vi "PID Control.vi"(0 "Set Point":cluster{"SetPoint X":dbl, "SetPoint Y":dbl}, 3 "Actual Value":cluster{"Actual X":dbl, "Actual Y":dbl}, 4 "PID Gain X":T1={"proportional gain (Kc)"=1.0, "integral time (Ti, min)"=0.01, "derivative time (Td, min)"=0.0} {"derivative time (Td, min)" format="%.3f"; "integral time (Ti, min)" format="%.3f"; "proportional gain (Kc)" format="%.3f"}, 5 "PID Gain Y":T1={"proportional gain (Kc)"=1.0, "integral time (Ti, min)"=0.01, "derivative time (Td, min)"=0.0} {"derivative time (Td, min)" format="%.3f"; "integral time (Ti, min)" format="%.3f"; "proportional gain (Kc)" format="%.3f"}) -> (7 "Output PID X":dbl format="%.2f", 10 "Output PID Y":dbl format="%.2f")   [LabVIEW 2015]
uses:
  <vilib>/addons/control/pid/pid.llb/PID (DBL).vi
  <vilib>/addons/control/pid/NI_PID_pid.lvlib
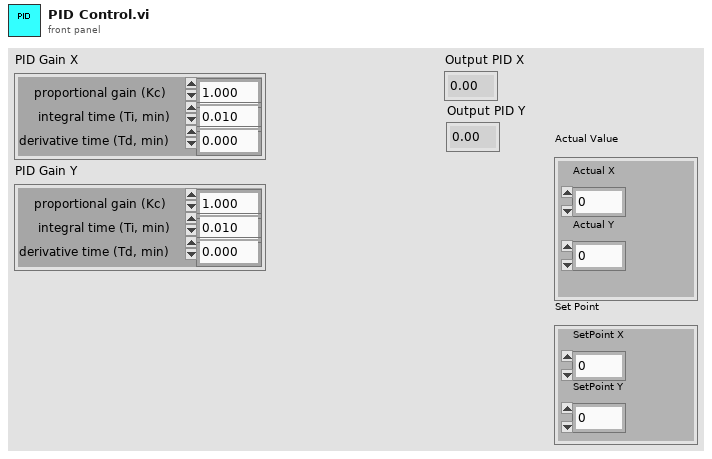
[diagram p1: front panel]
types:
  T1 = cluster{"proportional gain (Kc)":dbl, "integral time (Ti, min)":dbl, "derivative time (Td, min)":dbl}
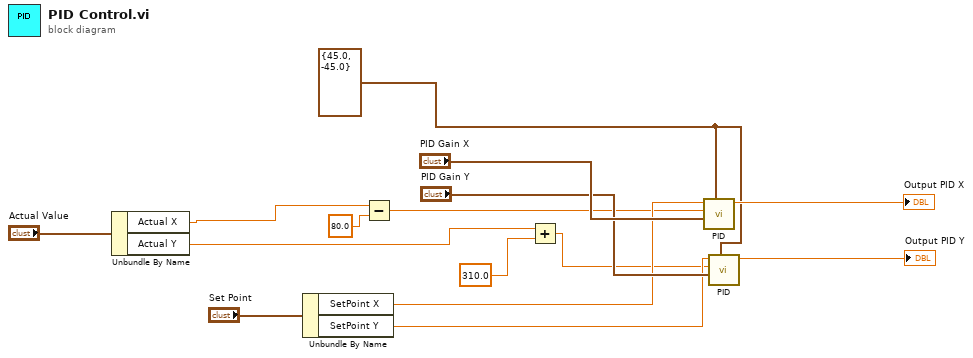
[diagram p0: block diagram]
diagram:
  w1 = cluster{dbl, dbl} {45.0, -45.0}
  n1 = Unbundle By Name("Actual Value") -> ("Actual X"=w7:dbl, "Actual Y"=w5:dbl)
  n2 = Unbundle By Name("Set Point") -> ("SetPoint X"=w11:dbl, "SetPoint Y"=w10:dbl)
  n3 = Subtract(x=w7, y=80.0) -> (x-y=w6:dbl)
  n4 = Add(x=w5, y=310.0) -> (x+y=w4:dbl)
  n5 = call-poly <vilib>:"PID.vi"("output range"=w1, "PID gains"="PID Gain X", "process variable"=w6, "setpoint"=w11) -> ("output"=→"Output PID X":dbl)  [unwired: 6 in, 1 out]
  n6 = call-poly <vilib>:"PID.vi"("output range"=w1, "PID gains"="PID Gain Y", "process variable"=w4, "setpoint"=w10) -> ("output"=→"Output PID Y":dbl)  [unwired: 6 in, 1 out]
